vi "Parse configuration.vi"(8 "error in (no error)":errorcluster, 9 "Mode Name for Variant":string[](array[string]), 10 "Config File Sections":string[](array[string]), 11 "Refnum in":T1) -> (0 "error out":errorcluster, 3 "Variant array":variant[](array[variant]))   [LabVIEW 2025]
doc: "Author: Scott Hannahs <sth@magnet.fsu.edu>\n\nThis software is licensed for use under the “MIT License\"\nCopyright (c) 2025 Scott Hannahs, sth@sth@magnet.sthnet.net\n\nPermission is hereby granted, free of charge, to any person obtaining a copy of this software and associated documentation files (the \"Software\"), to deal in the Software without restriction, including without limitation the rights to use, copy, modify, merge, publish, distribute, sublicense, and/or sell copies of the Software, and to permit persons to whom the Software is furnished to do so, subject to the following conditions: The above copyright notice and this permission notice shall be included in all copies or substantial portions of the Software.\n\nTHE SOFTWARE IS PROVIDED \"AS IS\", WITHOUT WARRANTY OF ANY KIND, EXPRESS OR IMPLIED, INCLUDING BUT NOT LIMITED TO THE WARRANTIES OF MERCHANTABILITY, FITNESS FOR A PARTICULAR PURPOSE AND NONINFRINGEMENT. IN NO EVENT SHALL THE AUTHORS OR COPYRIGHT HOLDERS BE LIABLE FOR ANY CLAIM, DAMAGES OR OTHER LIABILITY, WHETHER IN AN ACTION OF CONTRACT, TORT OR OTHERWISE, ARISING FROM, OUT OF OR IN CONNECTION WITH THE SOFTWARE OR THE USE OR OTHER DEALINGS IN THE SOFTWARE."
uses:
  <vilib>/Utility/config.llb/Config Data RefNum.ctl
  <vilib>/Utility/config.llb/Read Key (String).vi
  <vilib>/Utility/config.llb/NI_LVConfig.lvlib
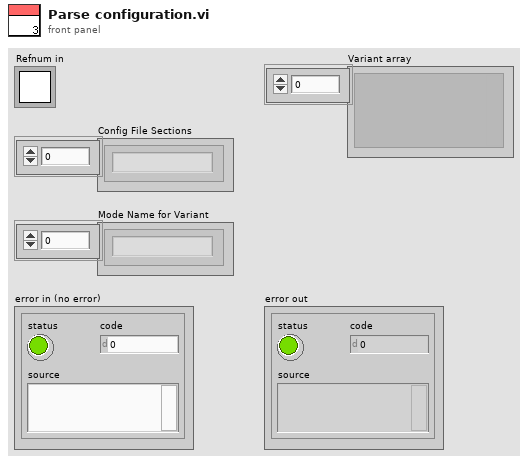
[diagram p1: front panel]
types:
  T1 = typedef "NI_LVConfig.lvlib/Config Data RefNum.ctl" = refnum<k1>
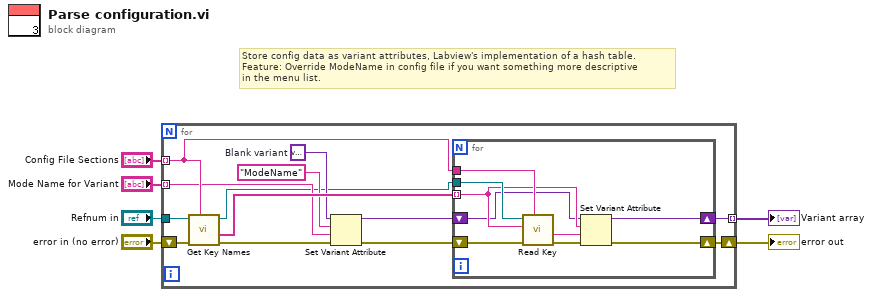
[diagram p0: block diagram]
diagram:
  # "Store config data as variant attributes, Labview's implementation of a hash table.\nFeature: Override ModeName in config file if you want something more descriptive\nin the menu list."
  n1 = for {
    shift-right: [w15] -> w6
    shift-left: "error in (no error)" -> [w19]
    tunnel: "Config File Sections" -> [w16] mode=indexing
    tunnel: "Refnum in" -> [w18]
    tunnel: "Mode Name for Variant" -> [w11] mode=indexing
    tunnel: [w14] -> w5 mode=indexing
    w12 = variant  # Blank variant
    n2 = call <vilib>:"Get Key Names.vi"("section"=w16, "error in (no error)"=w19, "refnum"=w18) -> ("error out"=w10:errorcluster, "key names"=w17:string[], "refnum out"=w9:T1)  [unwired: 5 in, 1 out]
    n3 = Set Variant Attribute(Variant=w12, name="ModeName", value=w11, error in=w10) -> (Variant out=w7:variant, error out=w8:errorcluster)  [unwired: 1 out]
    n4 = for {
      tunnel: w17 -> [w22] mode=indexing
      tunnel: w16 -> [w28]
      tunnel: w9 -> [w27]
      shift-right: [w24] -> w15
      shift-left: w8 -> [w26]
      shift-right: [w20] -> w14
      shift-left: w7 -> [w21]
      n5 = call-poly <vilib>:"Read Key.vi"("section"=w28, "error in (no error)"=w26, "key"=w22, "refnum"=w27) -> ("error out"=w25:errorcluster, "value"=w23:string)  [unwired: 4 in, 2 out]
      n6 = Set Variant Attribute(Variant=w21, name=w22, value=w23, error in=w25) -> (Variant out=w20:variant, error out=w24:errorcluster)  [unwired: 1 out]
    }
  }
  "error out" <- w6
  "Variant array" <- w5
